vi "Test Timeout.vi"(8 "error in (no error)":errorcluster) -> (0 "error out":errorcluster)   [LabVIEW 2020, in "TEST JKI State Machine API.lvlib"]
uses:
  TEST JKI State Machine API.lvlib
  source/JKI SM/JKI SM.lvclass
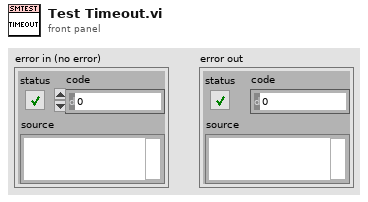
[diagram p1: front panel]
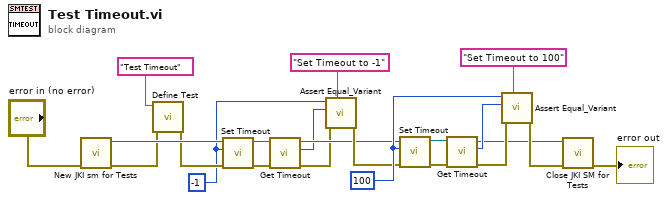
[diagram p0: block diagram]
diagram:
  w15 = 100 ("Timeout (ms)")
  w6 = -1 ("Timeout (ms)")
  n1 = call "New JKI sm for Tests.vi"("error in (no error)"="error in (no error)") -> ("error out"=w21:errorcluster, "JKI SM out"=w22:refnum<class "JKI SM.lvclass">)  [unwired: 9 in]
  n2 = call <vilib>:"Define Test.vi"("error in (no error)"=w21, "Label (VI Title)"="Test Timeout") -> ("error out"=w19:errorcluster)  [unwired: 8 in, 1 out]
  n3 = call "Set Timeout.vi"("error in (no error)"=w19, "Timeout (ms)"=w6, "JKI SM in"=w22) -> ("error out"=w4:errorcluster, "JKI SM out"=w5:refnum<class "JKI SM.lvclass">)  [unwired: 7 in]
  n4 = call "Get Timeout.vi"("error in (no error)"=w4, "JKI SM in"=w5) -> ("error out"=w11:errorcluster, "Timeout (ms)"=w7:i32, "JKI SM out"=w12:refnum<class "JKI SM.lvclass">)  [unwired: 7 in]
  n5 = call <vilib>:"Assert Equal_Variant.vi"("Label"="Set Timeout to -1", "error in (no error)"=w11, "Y"=w7, "X"=w6) -> ("error out"=w13:errorcluster)  [unwired: 7 in]
  n6 = call "Set Timeout.vi"("error in (no error)"=w13, "Timeout (ms)"=w15, "JKI SM in"=w12) -> ("error out"=w10:errorcluster, "JKI SM out"=w9:refnum<class "JKI SM.lvclass">)  [unwired: 7 in]
  n7 = call "Get Timeout.vi"("error in (no error)"=w10, "JKI SM in"=w9) -> ("error out"=w17:errorcluster, "Timeout (ms)"=w16:i32, "JKI SM out"=w1:refnum<class "JKI SM.lvclass">)  [unwired: 7 in]
  n8 = call <vilib>:"Assert Equal_Variant.vi"("Label"="Set Timeout to 100", "error in (no error)"=w17, "Y"=w16, "X"=w15) -> ("error out"=w3:errorcluster)  [unwired: 7 in]
  n9 = call "Close JKI SM for Tests.vi"("error in (no error)"=w3, "JKI SM in"=w1) -> ("error out"=→"error out":errorcluster)  [unwired: 9 in]
